vi "Get Double.vi"(8 "error in (no error)":errorcluster, 11 "DoubleMsg In":refnum<class "DoubleMsg.lvclass">) -> (0 "error out":errorcluster, 2 "Message Data":dbl, 3 "DoubleMsg Out":refnum<class "DoubleMsg.lvclass">)   [LabVIEW 2018, in "LapDog.Messaging.v3.NativeTypes.lvlib" / "DoubleMsg.lvclass"]
doc: "Returns the data contained in the message.\n\nThis method executes regardless of the error in state."
uses:
  DoubleMsg.lvclass
  DoubleMsg.lvclass/DoubleMsg.ctl
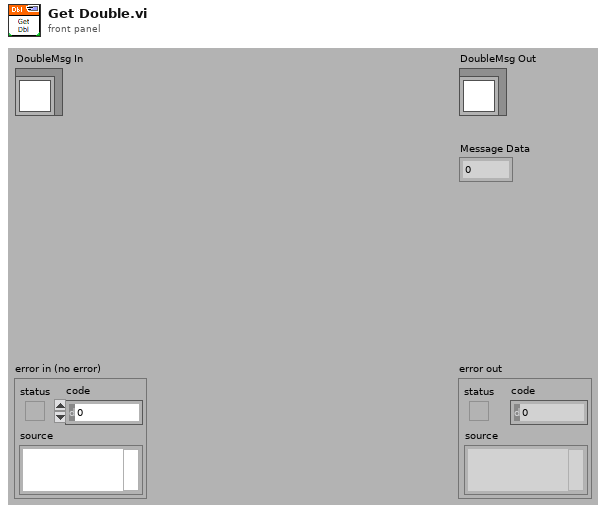
[diagram p1: front panel]
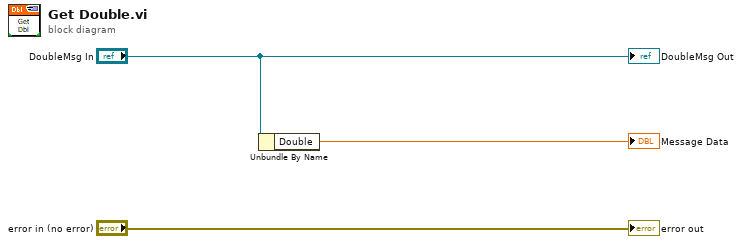
[diagram p0: block diagram]
diagram:
  n1 = Unbundle By Name("DoubleMsg In") -> ("Double"=→"Message Data":dbl)
  "error out" <- "error in (no error)"
  "DoubleMsg Out" <- "DoubleMsg In"
